vi "Motion Down.vi"(10 "Command":string) -> (2 "Motion Down":bool)   [LabVIEW 2017]
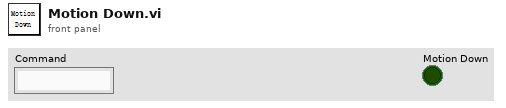
[diagram p1: front panel]
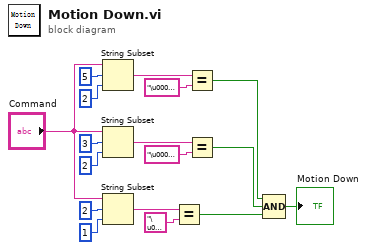
[diagram p0: block diagram]
diagram:
  n1 = String Subset(string="Command", offset (0)=5 ("偏移量(0)"), length (rest)=2 ("长度（剩余）")) -> (substring=w7:string)
  n2 = String Subset(string="Command", offset (0)=3 ("偏移量(0)"), length (rest)=2 ("长度（剩余）")) -> (substring=w5:string)
  n3 = String Subset(string="Command", offset (0)=2 ("偏移量(0)"), length (rest)=1 ("长度（剩余）")) -> (substring=w15:string)
  n4 = Equal?(x=w15, y="\u0004") -> (x = y?=w2:bool)
  n5 = Equal?(x=w7, y="\u0000\u0001" ("子字符串")) -> (x = y?=w4:bool)
  n6 = Equal?(x=w5, y="\u0000\u0000" ("子字符串 2")) -> (x = y?=w3:bool)
  n7 = Compound Arithmetic op=AND ("复合运算")(w4, w3, w2) -> (→"Motion Down":bool)
